vi "Get SysDef Target List.vi"(8 "error in (no error)":errorcluster, 11 "System Definition Path":path) -> (0 "error out":errorcluster, 2 "Target List":refnum<k24>[](array[refnum]))   [LabVIEW 2019, in "TLCD Test Class.lvclass"]
uses:
  TLCD Test Class.lvclass
  NationalInstruments.VeriStand.SystemDefinitionAPI
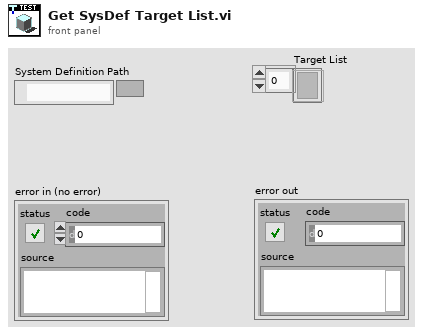
[diagram p1: front panel]
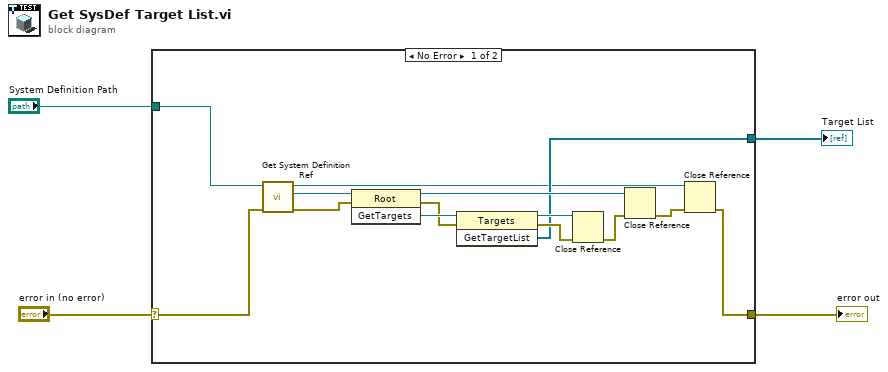
[diagram p0: block diagram]
diagram:
  n1 = case shown="No Error" "error in (no error)" {
    selector: "error in (no error)" -> [w9 w19]
    tunnel: "System Definition Path" -> [w10 _]
    tunnel: [w8 _] -> w2
    tunnel: [w5 w19] -> w1
    frame No Error {
      n2 = call "Get System Definition Ref.vi"("error in (no error)"=w9, "System Definition Path"=w10) -> ("error out"=w13:errorcluster, "System Definition Root Ref"=w12:refnum<k24>, "System Definition Ref"=w6:refnum<k24>)  [unwired: 7 in]
      n3 = invoke class="Root" method="GetTargets"(reference=w12, error in=w13) -> (reference out=w16:refnum<k24>, error out=w11:errorcluster, "GetTargets"=w14:refnum<k24>)  [unwired: 1 in]
      n4 = invoke class="Targets" method="GetTargetList"(reference=w14, error in=w11) -> (reference out=w17:refnum<k24>, error out=w18:errorcluster, "GetTargetList"=w8:refnum<k24>[])  [unwired: 1 in]
      n5 = Close Reference(reference=w17, error in (no error)=w18) -> (error out=w15:errorcluster)
      n6 = Close Reference(reference=w16, error in (no error)=w15) -> (error out=w7:errorcluster)
      n7 = Close Reference(reference=w6, error in (no error)=w7) -> (error out=w5:errorcluster)
    }
    frame Error {
    }
  }
  "Target List" <- w2
  "error out" <- w1
